vi "get all control details.vi"(8 "error in":errorcluster, 11 "VI (Caller)":refnum<vi>) -> (0 "error out":errorcluster, 3 "Control details":string)   [LabVIEW 2020, in "ui-testing.lvlib"]
uses:
  ui-testing.lvlib
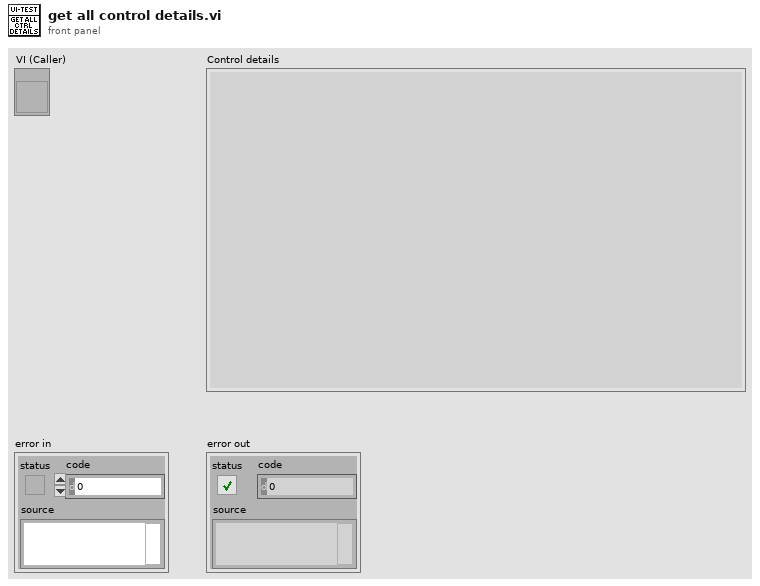
[diagram p1: front panel]
types:
  T1 = cluster{"Caption":string, "Label":string, "Visible":bool}
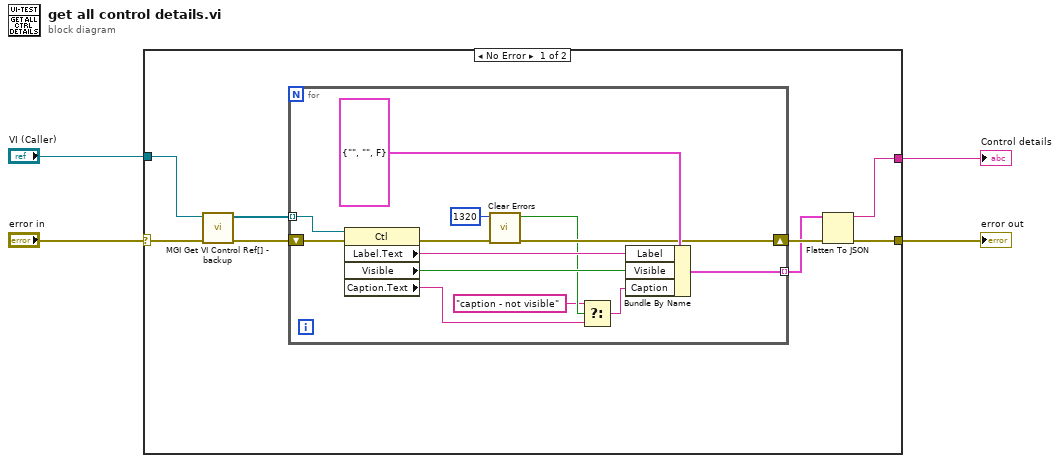
[diagram p0: block diagram]
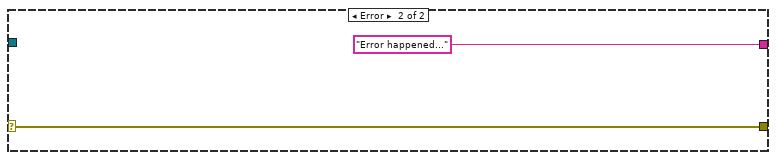
[diagram p2: hidden frame]
diagram:
  n1 = case shown="No Error" "error in" {
    selector: "error in" -> [w5 w27]
    tunnel: [w9 w27] -> w4
    tunnel: [w7 "Error happened..."] -> w3
    tunnel: "VI (Caller)" -> [w6 _]
    frame No Error {
      n2 = call "MGI Get VI Control Ref[] - backup.vi"("error in"=w5, "VI (Caller)"=w6) -> ("error out"=w12:errorcluster, "Control[i]"=w11:refnum<vi>[])  [unwired: 6 in, 2 out]
      n3 = for {
        tunnel: w11 -> [w24] mode=indexing
        tunnel: [w20] -> w8 mode=indexing
        shift-right: [w18] -> w10
        shift-left: w12 -> [w25]
        n4 = property class="Ctl"(reference=w24, error in=w25) -> (error out=w19:errorcluster, "Label.Text"=w23:string, "Visible"=w22:bool, "Caption.Text"=w16:string)  [unwired: 1 out]
        n5 = call <vilib>:"Clear Errors.vi"("error in (no error)"=w19, "specific error code to clear (0: all)"=1320) -> ("error out"=w18:errorcluster, "specific error cleared?"=w14:bool)  [unwired: 4 in]
        n6 = Select(t="caption - not visible", s=w14, f=w16) -> (s? t:f=w15:string)
        n7 = Bundle By Name(cluster=T1 {"Caption"="", "Label"="", "Visible"=FALSE}, "Label"=w23, "Visible"=w22, "Caption"=w15) -> (w20:T1)
      }
      n8 = Flatten To JSON(anything=w8, error in (no error)=w10) -> (JSON string=w7:string, 11:w9:errorcluster)  [unwired: 1 in]
    }
    frame Error {
    }
  }
  "error out" <- w4
  "Control details" <- w3
